vi "EOL CAN_Check Incoming Rx Length.vi"(8 "TxRx Data in":string[][](array[string]), 9 "Tx":u8[](array[numeric]), 10 "Rx Arbitration Id":u32, 11 "data":T1[](array[typedef]) {"payload" format="%x"; "timestamp" format="%<%.7X\n%x>T"; "type" items=["CAN Data"=0, "CAN Remote"=1, "CAN Bus Error"=2, "CAN 2.0 Data"=8, "CAN FD Data"=16, "CAN FD+BRS Data"=24, "J1939 Data"=192, "Delay"=224, "Log Trigger"=225, "Start Trigger"=226]; "identifier" format="%x"}) -> (0 "TxRx Data out":string[][](array[string]), 1 "Rx Bytes":u8, 2 "Rx Data":u8[](array[numeric]), 3 "Response Good?":bool)   [LabVIEW 2018]
uses:
  <vilib>/xnet/xnet.llb/XNET Frame CAN.ctl
  <vilib>/xnet/xnet.llb/XNET Frame Type CAN.ctl
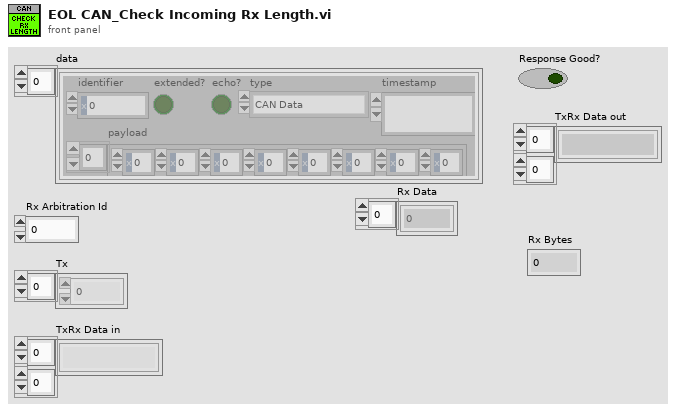
[diagram p1: front panel]
types:
  T1 = typedef "XNET Frame CAN.ctl" = cluster{"timestamp":timestamp, "payload":u8[], "identifier":u32, "type":T2, "extended?":bool, "echo?":bool}
  T2 = typedef "XNET Frame Type CAN.ctl" = u8
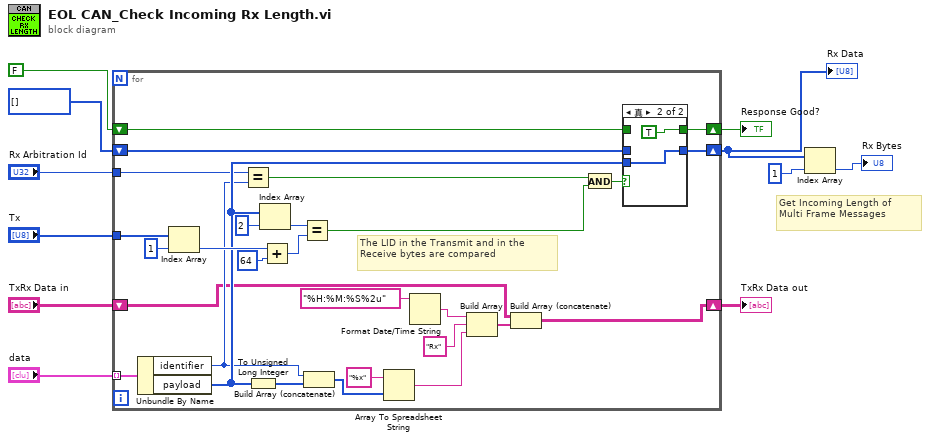
[diagram p0: block diagram]
diagram:
  # "Get Incoming Length of \nMulti Frame Messages"
  n1 = for {
    tunnel: "data" -> [w39] mode=indexing
    shift-right: [w38] -> w3
    shift-left: u8[] [] ("Data Array") -> [w37]
    shift-right: [w36] -> w11
    shift-left: FALSE -> [w35]
    tunnel: "Tx" -> [w29]
    shift-right: [w16] -> w6
    shift-left: "TxRx Data in" -> [w17]
    tunnel: "Rx Arbitration Id" -> [w14]
    # "The LID in the Transmit and in the\nReceive bytes are compared"
    n2 = Unbundle By Name(w39) -> ("identifier"=w22:u32, "payload"=w23:u8[])
    n3 = Index Array(array=w29, index=1) -> (element=w31:u8)
    n4 = Equal?(x=w14, y=w22) -> (x = y?=w33:bool)
    n5 = To Unsigned Long Integer(number=w23) -> (unsigned 32bit integer=w24:u32[])
    n6 = Index Array(array=w23, index=2) -> (element=w28:u8)
    n7 = Add(x=w31, y=u8 64 ("Numeric")) -> (x+y=w27:u8)
    n8 = Equal?(x=w28, y=w27) -> (x = y?=w26:bool)
    n9 = Build Array (concatenate)(w22, w24) -> (w15:u32[])
    n10 = Array To Spreadsheet String(array=w15, 3:"%x" ("format string")) -> (spreadsheet string=w19:string)  [unwired: 1 in]
    n11 = Format Date/Time String(time format string (%c)="%H:%M:%S%2u" ("时间格式字符串(%c)")) -> (date/time string=w13:string)  [unwired: 2 in]
    n12 = Build Array(w13, "Rx" ("format string"), w19) -> (w18:string[])
    n13 = Build Array (concatenate)(w17, w18) -> (w16:string[][])
    n14 = And(x=w33, y=w26) -> (x .and. y?=w34:bool)
    n15 = case shown="真" w34 {
      tunnel: w23 -> [_ w42]
      tunnel: [w41 w42] -> w38
      tunnel: w37 -> [w41 _]
      tunnel: [w40 TRUE] -> w36
      tunnel: w35 -> [w40 _]
      frame False {
      }
      frame True {
      }
    }
  }
  "Response Good?" <- w11
  "TxRx Data out" <- w6
  "Rx Data" <- w3
  n16 = Index Array(array=w3, index=1) -> (element=→"Rx Bytes":u8)
